vi "Divide Quaternion by Quaternion.vi"(1 "y":T1, 2 "quaternion":T1) -> (0 "quotient":T1)   [LabVIEW 2017, in "NI_Kinematics.lvlib"]
doc: "Computes the <B>quotient</B> of two quaternions or a quaternion and a scalar number. Wire data to the <B>y</B> input to determine the polymorphic instance to use or manually select the instance."
uses:
  <vilib>/robotics/Kinematics/NI_Kinematics.lvlib
  <vilib>/robotics/Kinematics/Quaternion.ctl
  <vilib>/Analysis/baseanly.llb/Dot Product.vi
  <vilib>/Analysis/baseanly.llb/Real Dot Product.vi
  <vilib>/robotics/Kinematics/Conjugate Quaternion.vi
  <vilib>/robotics/Kinematics/Multiply Quaternion by Quaternion.vi
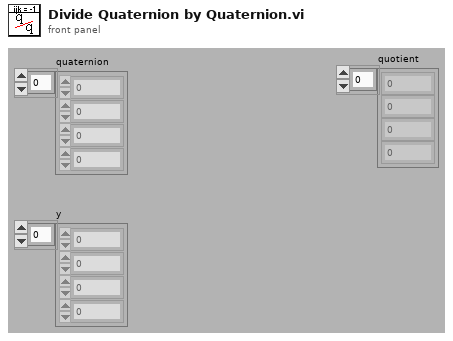
[diagram p1: front panel]
types:
  T1 = typedef "NI_Kinematics.lvlib/Quaternion.ctl" = dbl[]
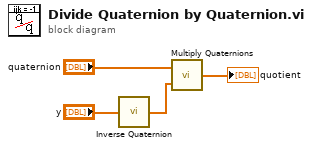
[diagram p0: block diagram]
diagram:
  n1 = call <vilib>:"Inverse Quaternion.vi"("quaternion"="y") -> ("inverse"=w4:T1)  [unwired: 1 in]
  n2 = call-poly <vilib>:"Multiply Quaternions.vi"("y"=w4, "quaternion"="quaternion") -> ("product"=→"quotient":T1)
